vi "custom_enqueue_states.vi"(7 "task":T1=[enum."(qsm) initialize"], 8 "error in":errorcluster, 11 "queue in":refnum<queue>) -> (0 "error out":errorcluster, 3 "queue out":refnum<queue>)   [LabVIEW 2017]
uses:
  type defs/states.ctl
  type defs/task.ctl
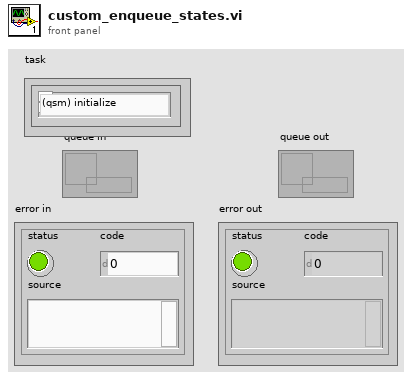
[diagram p1: front panel]
types:
  T1 = typedef "task.ctl" = T2[]
  T2 = typedef "states.ctl" = enum16{"(qsm) schedule", "(qsm) initialize", "(qsm) release", "(qsm) clean up", "(qsm) shutdown", "(myRIO) initialize", "(myRIO) clean up", "(myRIO) update ports", "(image) get", "(image) analyze", "(image) overlay", "(image) show", "save image", "(ball) Shape detection", "(ball) Calculate ROI", "X align", "Y align", "Wait", "Grab", "(pattern) Find Square", "(pattern) Calculate ROI", "(pattern) Analyze pattern", "Compare", "Wait for button"}
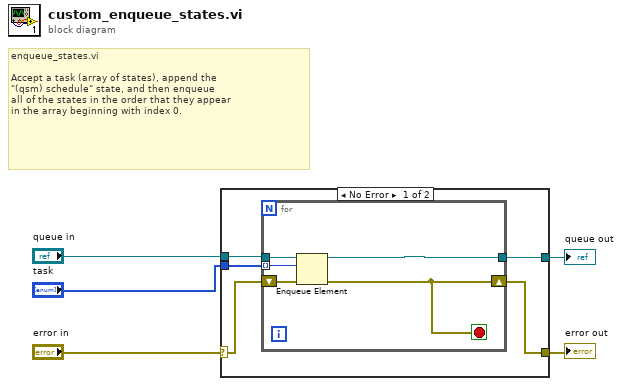
[diagram p0: block diagram]
diagram:
  # "enqueue_states.vi\n\nAccept a task (array of states), append the\n\"(qsm) schedule\" state, and then enqueue\nall of the states in the order that they appear\nin the array beginning with index 0."
  n1 = case shown="No Error" "error in" {
    selector: "error in" -> [w8 w17]
    tunnel: [w7 w17] -> w4
    tunnel: "queue in" -> [w10 w16]
    tunnel: [w9 w16] -> w2
    tunnel: "task" -> [w6 _]
    frame No Error {
      n2 = for {
        shift-right: [w12] -> w7
        shift-left: w8 -> [w15]
        tunnel: w10 -> [w14]
        tunnel: w6 -> [w13] mode=indexing
        tunnel: [w11] -> w9
        stop <- w12 stop-if-true
        n3 = Enqueue Element(queue=w14, element=w13, error in (no error)=w15) -> (queue out=w11:refnum<queue>, error out=w12:errorcluster)  [unwired: 1 in, 1 out]
      }
    }
    frame Error {
    }
  }
  "queue out" <- w2
  "error out" <- w4
